vi "GUI_laptop v6.vi"() -> ()   [LabVIEW 2019]
uses:
  <vilib>/Math Plots/3D Math Plots/3D Scatter/3D Scatter XCtrl/3D Scatter.xctl
  <vilib>/Platform/TimedLoop/XDataNode/timing_clust.ctl
  <vilib>/Platform/TimedLoop/XDataNode/nitl_modes.ctl
  <vilib>/Platform/TimedLoop/XDataNode/wakeup.ctl
  <vilib>/Analysis/_algsub.llb/Real Vector Norm.vi
  <vilib>/Instr/_visa.llb/VISA Configure Serial Port (Instr).vi
  <vilib>/Utility/file.llb/Write Delimited Spreadsheet (DBL).vi
  <vilib>/Math Plots/3D Math Plots/3D Scatter/3D Scatter Datatype/Public/Plot Helper (Vector).vi
  <vilib>/platform/TimedLoop/XDataNode/XDataNode.xnode
  <vilib>/Platform/TimedLoop/XDataNode/XDNodeRunTimeDep.lvlib
  <vilib>/Analysis/NI_AALPro.lvlib
  <vilib>/Math Plots/3D Math Plots/3D Scatter/3D Scatter Datatype/3D Scatter Datatype.lvclass
panel:
  out "send values":dbl[](array[numeric])
  in  "UDP Send":bool
  in  "UDP Recv":bool
  in  "L5 bound":dbl=1000.0
  in  "L4 bound (deg)":dbl=1000.0
  in  "L3 bound (mm)":dbl=1000.0
  in  "L2 bound (deg)":dbl=1000.0
  in  "L1 bound (deg)":dbl=1000.0
  in  "Joystick Type":dbl(ring) items=["Rigid Joystick", "Free Joystick"]
  out "Finished Late? [i-1]":bool
  in  "Epsilon":dbl=0.2
  out "3D Scatter":refnum<class "3D Plot Datatype.lvclass">[](xcontrol)
  out "Random Point":dbl[](array[numeric])
  out "Virtual Cursor":dbl[](array[numeric])
  out "Iteration Duration":i64
  in  "Num of Points":i32=10
  in  "z bound":dbl=2.0
  in  "y bound":dbl=5.0
  in  "x bound":dbl=5.0
  in  "Stop":bool
  in  "Round Decimals":dbl=2.0 format="%#_15g"
  in  "Save  Data":bool
  in  "Save Path":path
  in  "x speed":dbl=0.5
  in  "z speed":dbl=0.5
  in  "y speed":dbl=0.5
  out "error out":errorcluster
  in  "baud rate":u32=115200
  in  "VISA resource name":refnum<visa-resource-name>
  # "TODO: fix the bounds; currently bounds are arbitrary"
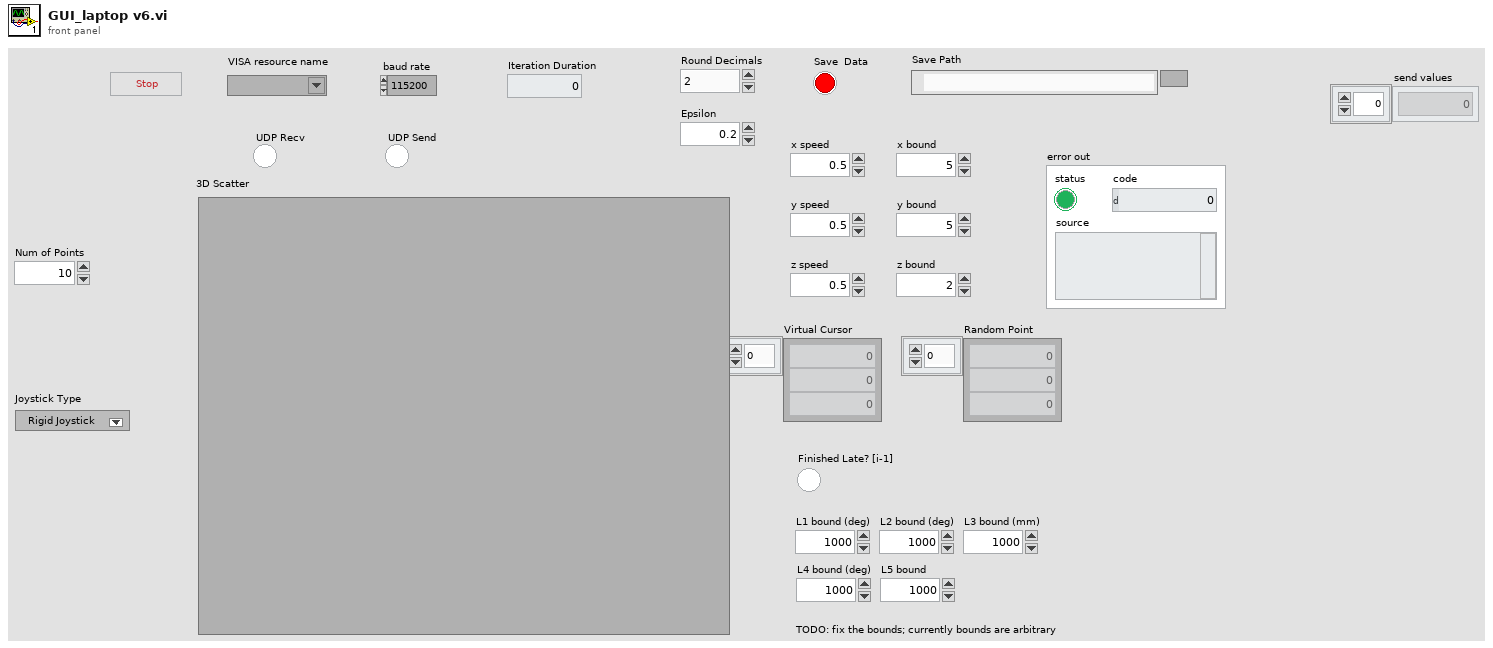
[diagram p1: front panel]
types:
  T1 = typedef "XDNodeRunTimeDep.lvlib/timing_clust.ctl" = cluster{"Expected End [f-1]":u64, "Actual End [f-1]":u64, "Finished Late? [f-1]":bool, "Expected End [i-1]":u64, "Actual End [i-1]":u64, "Finished Late? [i-1]":bool, "Expected Start [i]":u64, "Actual Start [i]":u64, "Expected Start [f]":u64, "Actual Start [f]":u64, "Source Name":string, "Structure Name":string, "Period":i64, "Deadline":i64, "Offset":i64, "Start":i64, "Priority":i32, "Timeout":i32, "Mode":T2, "Wakeup Reason":T3, "Error":errorcluster, "Source Type":string, "Secondary Source Type":string, "Global End Time":u64, "Global Start Time":u64, "Frame Duration":u64, "Iteration Duration":u64, "Assigned CPU":i32, "I/O Scan Engine Mode":u32}
  T2 = typedef "XDNodeRunTimeDep.lvlib/nitl_modes.ctl" = enum32{"No Change", "Process missed periods, maintain original phase", "Discard missed periods, maintain original phase", "Process missed periods, ignore original phase", "Discard missed periods, ignore original phase"}
  T3 = typedef "XDNodeRunTimeDep.lvlib/wakeup.ctl" = enum32{"Normal", "Aborted", "Asynchronous wakeup", "Timing source error", "Timed loop error", "Timeout"}
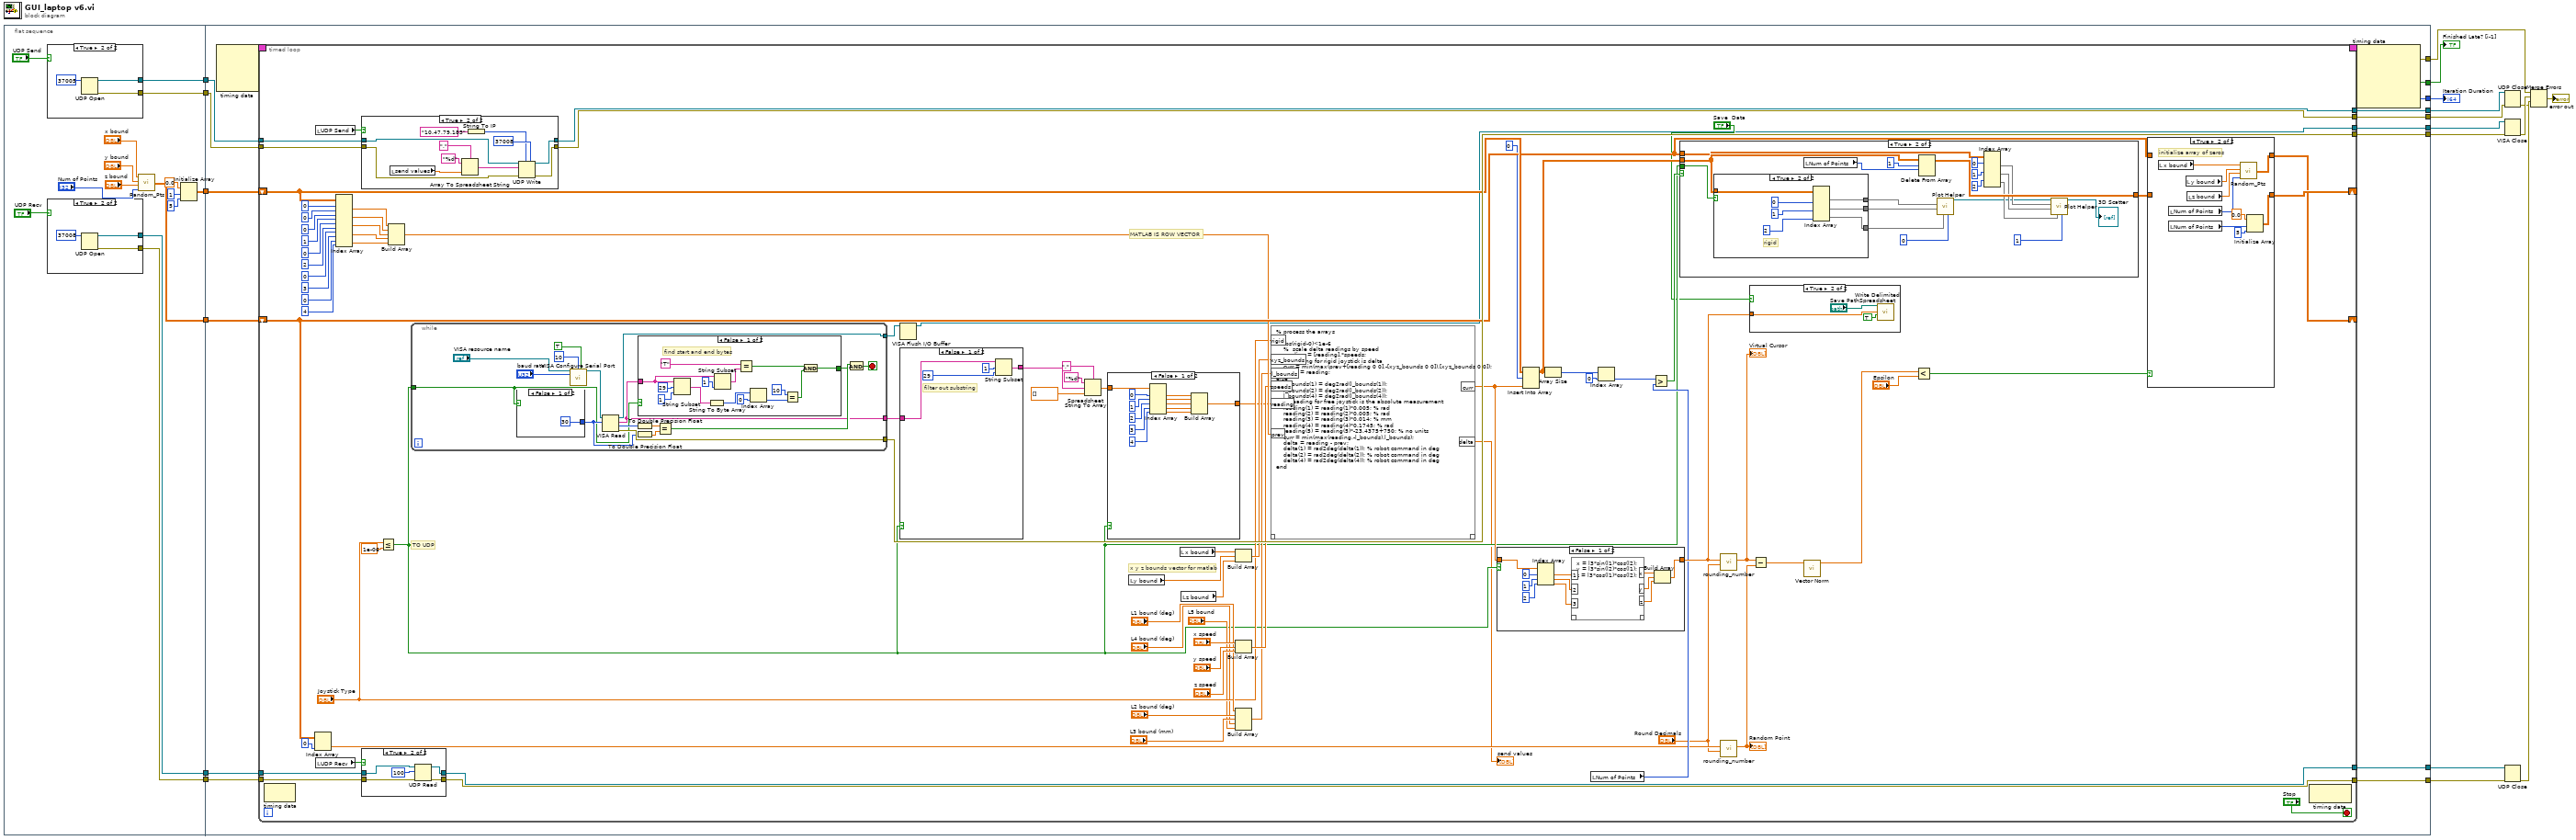
[diagram p0: block diagram]
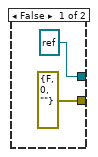
[diagram p2: hidden frame]
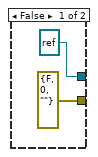
[diagram p3: hidden frame]
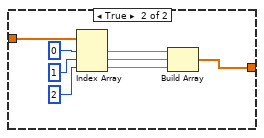
[diagram p9: hidden frame]
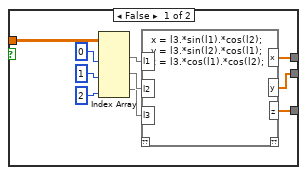
[diagram p12: hidden frame]
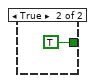
[diagram p13: hidden frame]
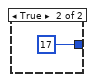
[diagram p14: hidden frame]
diagram:
  n1 = flat-sequence {
    tunnel: [w26] -> w15
    tunnel: [w30] -> w14
    tunnel: [w25] -> w13
    tunnel: [w24] -> w12
    tunnel: [w21] -> w11
    tunnel: [w20] -> w10
    tunnel: [w59] -> w19
    tunnel: [w58] -> w18
    tunnel: [w56] -> w9
    tunnel: [w54] -> w17
    tunnel: [w53] -> w16
    tunnel: w15 -> [w57]
    tunnel: w14 -> [w55]
    tunnel: w13 -> [w52]
    tunnel: w12 -> [w51]
    tunnel: w11 -> [w50]
    tunnel: w10 -> [w49]
    tunnel: [w48] -> w3
    tunnel: [w47] -> w8
    tunnel: [w46] -> w2
    tunnel: [w45] -> w1
    frame #0 {
      n2 = case shown="True" "UDP Send" {
        tunnel: [refnum<k16> refnum ("port") w38] -> w25
        tunnel: [errorcluster {"status"=FALSE, "code"=0, "source"=""} ("error out") w37] -> w20
        frame False {
        }
        frame True {
          n3 = UDP Open(11:u16 37005 ("port")) -> (port=w38:refnum<k16>, 0:w37:errorcluster)  [unwired: 4 in, 1 out]
        }
      }
      n4 = case shown="True" "UDP Recv" {
        tunnel: [refnum<k16> refnum ("port") w43] -> w24
        tunnel: [errorcluster {"status"=FALSE, "code"=0, "source"=""} ("error out") w42] -> w21
        frame False {
        }
        frame True {
          n5 = UDP Open(11:u16 37008 ("port")) -> (port=w43:refnum<k16>, 0:w42:errorcluster)  [unwired: 4 in, 1 out]
        }
      }
      n6 = call "Random_Pts.vi"("Num of Points"="Num of Points", "z bound"="z bound", "y bound"="y bound", "x bound"="x bound") -> ("appended array"=w30:dbl[][])
      n7 = Initialize Array(0.0 ("element"), 1 ("dimension size"), 5 ("dimension size")) -> (w26:dbl[][])
    }
    frame #1 {
      n8 = node-c288() -> (w61:T1)  [unwired: 4 in]
      n9 = timed-loop {
        tunnel: [w73] -> w59
        tunnel: [w139] -> w58
        shift-right: [w138] -> _
        shift-left: w57 -> [w137]
        timing: w61 -> [_]
        timing-out: [_] -> w60
        shift-right: [w133] -> _
        shift-left: w55 -> [w134]
        tunnel: w52 -> [w72]
        tunnel: w51 -> [w71]
        tunnel: w50 -> [w69]
        tunnel: w49 -> [w67]
        tunnel: [w66] -> w48
        tunnel: [w65] -> w47
        tunnel: [w64] -> w46
        tunnel: [w63] -> w45
        stop <- "Stop" stop-if-true
        # "TO UDP"
        # "MATLAB IS ROW VECTOR"
        # "x y z bounds vector for matlab"
        n10 = node-c288() -> ()  [unwired: 1 in, 1 out]
        n11 = Index Array(array=w134, index (col)=0 ("index (row)")) -> (element=w84:dbl[])  [unwired: 1 in]
        n12 = local read "UDP Send"() -> (w68:bool)
        n13 = local read "UDP Recv"() -> (w70:bool)
        n14 = Index Array(array=w137, index (row) #1=0 ("disabled index (row)"), index (col) #1=0 ("disabled index (col)"), index (row) #2=0 ("disabled index (row)"), index (col) #2=1 ("disabled index (col)"), index (row) #3=0 ("disabled index (row)"), index (col) #3=2 ("disabled index (col)"), index (row) #4=0 ("disabled index (row)"), index (col) #4=3 ("disabled index (col)"), index (row) #5=0 ("disabled index (row)"), index (col) #5=4 ("disabled index (col)")) -> (element #1=w110:dbl, element #2=w109:dbl, element #3=w108:dbl, element #4=w93:dbl, element #5=w92:dbl)
        n15 = case shown="True" w68 {
          tunnel: w72 -> [w141 w153]
          tunnel: w67 -> [w142 w148]
          tunnel: [w142 w144] -> w65
          tunnel: [w141 w143] -> w63
          frame False {
          }
          frame True {
            n16 = local read "send values"() -> (w152:dbl[])
            n17 = Array To Spreadsheet String(delimiter (Tab)=",", array=w152, 3:"%d" ("format string")) -> (spreadsheet string=w149:string)
            n18 = String To IP(1:"10.47.79.183" ("name")) -> (0:w146:u32)
            n19 = UDP Write(address=w146, port or service name=u16 37008, connection ID=w153, data in=w149, 8:w148) -> (error out=w144:errorcluster, 3:w143:refnum<k16>)  [unwired: 1 in]
          }
        }
        n20 = case shown="True" w70 {
          tunnel: w71 -> [w154 w160]
          tunnel: w69 -> [w155 w159]
          tunnel: [w155 w158] -> w66
          tunnel: [w154 w157] -> w64
          frame False {
          }
          frame True {
            n21 = UDP Read(connection ID=w160, max size (548)=100, 8:w159) -> (error out=w158:errorcluster, 3:w157:refnum<k16>)  [unwired: 1 in, 3 out]
          }
        }
        n22 = Less Or Equal?(x="Joystick Type", y=1e-06) -> (x <= y?=w86:bool)
        n23 = Build Array(w110, w109, w108, w93, w92) -> (w107:dbl[])
        n24 = while {
          tunnel: [w249] -> w87
          tunnel: [w262] -> w139
          tunnel: [w256] -> w74
          tunnel: w86 -> [w250]
          stop <- w252 stop-if-true
          n25 = case shown="False" w250 {
            tunnel: [30 u32 17 ("byte count")] -> w255
            frame False {
            }
            frame True {
            }
          }
          n26 = call-poly "VISA Configure Serial Port"("VISA resource name"="VISA resource name", "termination char\n(0xA = '\\n' = LF)"=u8 10 ("termination char\n(0xA = '\\n' = LF)"), "Enable Termination\nChar (T)"=TRUE ("Enable Termination\nChar (T)"), "baud rate (9600)"="baud rate") -> ("VISA resource name out"=w257:refnum<visa-resource-name>)  [unwired: 10 in, 1 out]
          n27 = VISA Read(VISA resource name=w257, byte count=w255) -> (VISA resource name out=w256:refnum<visa-resource-name>, read buffer=w249:string, return count=w264:u32, error out=w262:errorcluster)  [unwired: 1 in]
          n28 = To Double Precision Float(number=w264) -> (double precision float=w263:dbl)
          n29 = To Double Precision Float(number=w255) -> (double precision float=w254:dbl)
          n30 = case shown="False" w250 {
            tunnel: [w271 TRUE] -> w251
            tunnel: w249 -> [w274 _]
            frame False {
              # "find start and end bytes"
              n31 = String Subset(string=w274, offset (0)=29, length (rest)=1) -> (substring=w269:string)
              n32 = String To Byte Array(string=w269) -> (unsigned byte array=w268:u8[])
              n33 = String Subset(string=w274, length (rest)=1) -> (substring=w277:string)  [unwired: 1 in]
              n34 = Equal?(x="T", y=w277) -> (x = y?=w273:bool)
              n35 = Index Array(array=w268, index=0) -> (element=w266:u8)
              n36 = Equal?(x=10, y=w266) -> (x = y?=w272:bool)
              n37 = And(x=w273, y=w272) -> (x .and. y?=w271:bool)
            }
            frame True {
            }
          }
          n38 = Equal?(x=w263, y=w254) -> (x = y?=w253:bool)
          n39 = And(x=w253, y=w251) -> (x .and. y?=w252:bool)
        }
        n40 = VISA Flush I/O Buffer(VISA resource name=w74) -> (VISA resource name out=w73:refnum<visa-resource-name>)  [unwired: 2 in, 1 out]
        n41 = case shown="False" w86 {
          tunnel: w87 -> [w178 w179]
          tunnel: [w175 w179] -> w85
          frame False {
            # "filter out substring"
            n42 = String Subset(string=w178, offset (0)=1, length (rest)=29) -> (substring=w175:string)
          }
          frame True {
          }
        }
        n43 = Spreadsheet String To Array(delimiter (Tab)=",", format string="%d", spreadsheet string=w85, array type (2D Dbl)=dbl[] []) -> (array=w89:dbl[])
        n44 = case shown="False" w86 {
          tunnel: w89 -> [w180 w193]
          tunnel: [w185 w192] -> w88
          frame False {
            n45 = Index Array(array=w180, index #1=0 ("Plot ID"), index #2=1 ("Plot ID"), index #3=2 ("Plot ID"), index #4=3 ("Plot ID"), index #5=4 ("Plot ID")) -> (element #1=w188:dbl, element #2=w187:dbl, element #3=w186:dbl, element #4=w182:dbl, element #5=w181:dbl)
            n46 = Build Array(w188, w187, w186, w182, w181) -> (w185:dbl[])
          }
          frame True {
            n47 = Index Array(array=w193, index #1=0 ("Plot ID"), index #2=1 ("Plot ID"), index #3=2 ("Plot ID")) -> (element #1=w196:dbl, element #2=w195:dbl, element #3=w194:dbl)
            n48 = Build Array(w196, w195, w194) -> (w192:dbl[])
          }
        }
        n49 = local read "y bound"() -> (w112:dbl)
        n50 = local read "x bound"() -> (w113:dbl)
        n51 = local read "z bound"() -> (w111:dbl)
        n52 = Build Array(w113, w112, w111) -> (w105:dbl[])
        n53 = Build Array("x speed", "y speed", "z speed") -> (w106:dbl[])
        n54 = Build Array("L1 bound (deg)", "L2 bound (deg)", "L3 bound (mm)", "L4 bound (deg)", "L5 bound") -> (w101:dbl[])
        n55 = script code="% process the arrays\n\nif abs(rigid-0)<1e-6\n    %  scale delta readings by speed\n    reading = [reading].*speeds;\n    % reading for rigid joystick is delta\n    curr = min(max(prev+[reading 0 0],-[xyz_bounds 0 0]),[xyz_bounds 0 0]);\n    delta = reading;\nelse\n    l_bounds(1) = deg2rad(l_bounds(1));\n    l_bounds(2) = deg2rad(l_bounds(2));\n    l_bounds(4) = deg2rad(l_bounds(4));\n    % reading for free joystick is the absolute measurement\n    reading(1) = reading(1)*0.005; % rad\n    reading(2) = reading(2)*0.005; % rad\n    reading(3) = reading(3)*0.014; % mm\n    reading(4) = reading(4)*0.1745; % rad\n    reading(5) = reading(5)*-23.4375+750; % no units\n    curr = min(max(reading,-l_bounds),l_bounds);\n    delta = reading - prev;\n    delta(1) = rad2deg(delta(1)); % robot command in deg\n    delta(2) = rad2deg(delta(2)); % robot command in deg\n    delta(4) = rad2deg(delta(4)); % robot command in deg\nend"("xyz_bounds"=w105, "speeds"=w106, "reading"=w88, "prev"=w107, "rigid"="Joystick Type", "l_bounds"=w101) -> ("curr"=w98:dbl[], "delta"=→"send values":dbl[])  [unwired: 1 in, 1 out]
        n56 = case shown="False" w86 {
          tunnel: w98 -> [w207 w211]
          tunnel: [w200 w211] -> w135
          frame False {
            n57 = Index Array(array=w207, index #1=0 ("Plot ID"), index #2=1 ("Plot ID"), index #3=2 ("Plot ID")) -> (element #1=w206:dbl, element #2=w205:dbl, element #3=w204:dbl)
            n58 = script code="x = l3*sin(l1)*cos(l2);\ny = l3*sin(l2)*cos(l1);\nz = l3*cos(l1)*cos(l2);"("l1"=w206, "l2"=w205, "l3"=w204) -> ("x"=w203:dbl, "y"=w202:dbl, "z"=w201:dbl)  [unwired: 1 in, 1 out]
            n59 = Build Array(w203, w202, w201) -> (w200:dbl[])
          }
          frame True {
          }
        }
        n60 = Insert Into Array(array=w137, index (row)=0, new element=w98) -> (w118:dbl[][])  [unwired: 1 in]
        n61 = Array Size(array=w118) -> (size(s)=w120:i32[])
        n62 = local read "Num of Points"() -> (w119:i32)
        n63 = Index Array(array=w120, index=0) -> (element=w121:i32)
        n64 = Greater?(x=w121, y=w119) -> (0:w117:bool)
        n65 = case shown="True" w117 {
          tunnel: w118 -> [w212 w230]
          tunnel: [w212 w229] -> w136
          tunnel: w134 -> [_ w228]
          tunnel: w86 -> [_ w213]
          frame False {
          }
          frame True {
            n66 = case shown="True" w213 {
              tunnel: w230 -> [w241 w245]
              tunnel: [w232 w244] -> w219
              tunnel: [w233 w243] -> w218
              tunnel: [w234 w242] -> w217
              frame False {
                n67 = Index Array(array=w241, index (col) #1=0 ("Plot ID"), index (col) #2=1 ("Plot ID"), index (col) #3=2 ("Plot ID")) -> (element #1=w237:dbl[], element #2=w236:dbl[], element #3=w235:dbl[])  [unwired: 3 in]
                n68 = script code="x = l3.*sin(l1).*cos(l2);\ny = l3.*sin(l2).*cos(l1);\nz = l3.*cos(l1).*cos(l2);"("l1"=w237, "l2"=w236, "l3"=w235) -> ("x"=w232:dbl[], "y"=w233:dbl[], "z"=w234:dbl[])  [unwired: 1 in, 1 out]
              }
              frame True {
                # "rigid"
                n69 = Index Array(array=w245, index (col) #1=0 ("disabled index (col)"), index (col) #2=1 ("index (col)"), index (col) #3=2 ("index (col)")) -> (element #1=w244:dbl[], element #2=w243:dbl[], element #3=w242:dbl[])  [unwired: 3 in]
              }
            }
            n70 = local read "Num of Points"() -> (w227:i32)
            n71 = Delete From Array(array=w230, length=1, index (row)=w227) -> (array with subset deleted=w229:dbl[][])  [unwired: 1 in, 1 out]
            n72 = call-poly <vilib>:"Plot Helper.vi"("Plot ID"=0, "z vector"=w217, "y vector"=w218, "x vector"=w219) -> ("3D Plot lvclass Array out"=w221:refnum<class "3D Plot Datatype.lvclass">[])  [unwired: 2 in, 5 out]
            n73 = Index Array(array=w228, index (row) #1=0 ("index (row)"), index (row) #2=1 ("index (row)"), index (row) #3=2 ("index (row)")) -> (element #1=w225:dbl[], element #2=w224:dbl[], element #3=w223:dbl[])  [unwired: 3 in]
            n74 = call-poly <vilib>:"Plot Helper.vi"("Plot ID"=1, "z vector"=w223, "y vector"=w224, "x vector"=w225, "3D Plot lvclass Array in"=w221) -> ("3D Plot lvclass Array out"=→"3D Scatter":refnum<class "3D Plot Datatype.lvclass">[])  [unwired: 1 in, 5 out]
          }
        }
        n75 = call "rounding_number.vi"("power of ten"="Round Decimals", "Array"=w135) -> ("rounded"=w81:dbl[])  [unwired: 9 in]
        "Virtual Cursor" <- w81
        n76 = call "rounding_number.vi"("power of ten"="Round Decimals", "Array"=w84) -> ("rounded"=w80:dbl[])  [unwired: 9 in]
        "Random Point" <- w80
        n77 = case shown="True" "Save  Data" {
          tunnel: w135 -> [_ w161]
          frame False {
          }
          frame True {
            n78 = call-poly <vilib>:"Write Delimited Spreadsheet.vi"("file path (dialog if empty)"="Save Path", "1D data"=w161, "append to file? (new file:F)"=TRUE) -> ()  [unwired: 11 in, 2 out]
          }
        }
        n79 = Subtract(x=w81, y=w80) -> (x-y=w79:dbl[])
        n80 = call-poly <vilib>:"Vector Norm.vi"("Input Vector"=w79) -> ("norm"=w78:dbl)  [unwired: 9 in, 1 out]
        n81 = Less?(x=w78, y="Epsilon") -> (x < y?=w76:bool)
        n82 = case shown="True" w76 {
          tunnel: w134 -> [w165 _]
          tunnel: [w165 w170] -> w133
          tunnel: w136 -> [w164 _]
          tunnel: [w164 w166] -> w138
          frame False {
          }
          frame True {
            # "initialize array of zeros"
            n83 = local read "x bound"() -> (w174:dbl)
            n84 = local read "Num of Points"() -> (w171:i32)
            n85 = local read "Num of Points"() -> (w168:i32)
            n86 = local read "y bound"() -> (w173:dbl)
            n87 = local read "z bound"() -> (w172:dbl)
            n88 = call "Random_Pts.vi"("Num of Points"=w171, "z bound"=w172, "y bound"=w173, "x bound"=w174) -> ("appended array"=w170:dbl[][])
            n89 = Initialize Array(0.0 ("element"), w168, 5 ("dimension size")) -> (w166:dbl[][])
          }
        }
        n90 = node-c288() -> ()  [unwired: 1 in, 1 out]
      }
      n91 = node-c288(w60) -> (w56:errorcluster, w53:bool, w54:i64)  [unwired: 3 out]
    }
  }
  n92 = UDP Close(connection ID=w1, 8:w8) -> (error out=w5:errorcluster)  [unwired: 1 out]
  n93 = VISA Close(VISA resource name=w19, error in (no error)=w18) -> (error out=w7:errorcluster)
  n94 = UDP Close(connection ID=w2, 8:w3) -> (error out=w6:errorcluster)  [unwired: 1 out]
  n95 = Merge Errors(w9, w7, w6, w5) -> (→"error out":errorcluster)
  "Iteration Duration" <- w17
  "Finished Late? [i-1]" <- w16
